vi "getConfig.vi"(8 "error in (no error)":errorcluster, 11 "DDSOutput in":refnum<class "DDSOutput.lvclass">) -> (0 "error out":errorcluster, 2 "Config":T1, 3 "DDSOutput out":refnum<class "DDSOutput.lvclass">)   [LabVIEW 2009, in "Hardware.lvlib" / "Channels.lvlib" / "DDSOutput.lvclass"]
uses:
  DDSOutput.lvclass
  DDSOutput.lvclass/DDSOutput.ctl
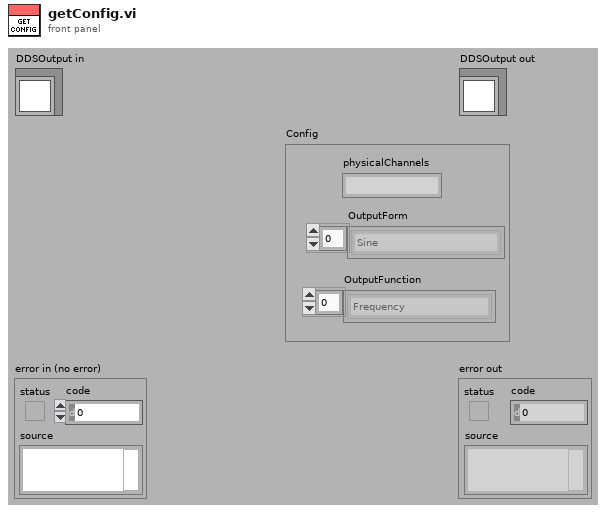
[diagram p1: front panel]
types:
  T1 = cluster{"OutputForm":enum16{"Sine", "Square", "Triangle", "Arbitrary"}[], "OutputFunction":enum16{"Frequency", "Ramp", "Sequence"}[], "physicalChannels":string}
  T2 = enum16{"Sine", "Square", "Triangle", "Arbitrary"}[]
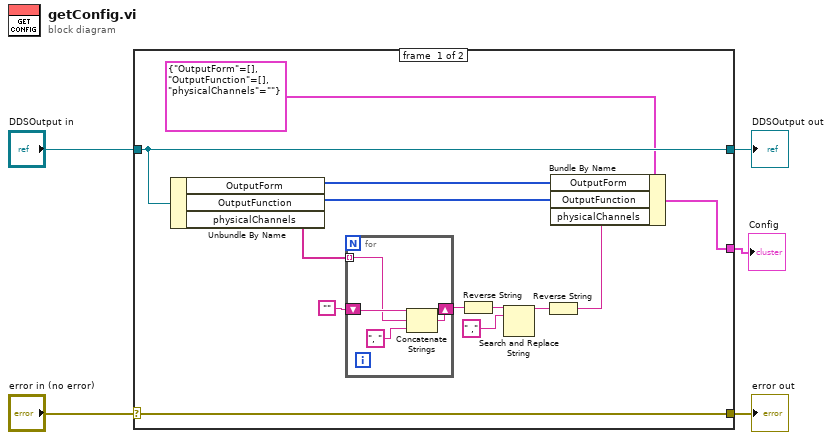
[diagram p0: block diagram]
diagram:
  n1 = case shown="No Error" "error in (no error)" {
    selector: "error in (no error)" -> [w18 w24]
    tunnel: [w18 w24] -> w4
    tunnel: [w17 w23] -> w2
    tunnel: "DDSOutput in" -> [w17 w23]
    tunnel: [w6 _] -> w1
    frame #0 {
      n2 = Unbundle By Name(w17) -> ("OutputForm"=w9:T2, "OutputFunction"=w8:enum16{"Frequency", "Ramp", "Sequence"}[], "physicalChannels"=w16:string[])
      n3 = for {
        tunnel: w16 -> [w21] mode=indexing
        shift-right: [w19] -> w14
        shift-left: "" -> [w22]
        n4 = Concatenate Strings(w22, w21, ", ") -> (w19:string)
      }
      n5 = Reverse String(1:w14) -> (0:w13:string)
      n6 = Search and Replace String(input string=w13, search string=" ,") -> (result string=w11:string)  [unwired: 6 in, 3 out]
      n7 = Reverse String(1:w11) -> (0:w7:string)
      n8 = Bundle By Name(cluster=T1 {"OutputForm"=[], "OutputFunction"=[], "physicalChannels"=""} ("Config"), "OutputForm"=w9, "OutputFunction"=w8, "physicalChannels"=w7) -> (w6:T1)
    }
    frame #1 {
    }
  }
  "error out" <- w4
  "DDSOutput out" <- w2
  "Config" <- w1
